vi "Igor_multi_singleXmultiY_ITX.vi"(1 "message":string, 2 "x-column name":string="field", 3 "graph file":cluster{"all rows":dbl[], "all rows":dbl[]}[](array[cluster])=[{"all rows"=array[1831 elements], "all rows"=array[1831 elements]}, {"all rows"=array[1238 elements], "all rows"=array[1238 elements]}, {"all rows"=array[1485 elements], "all rows"=array[1485 elements]}] {"all rows" format="%.2e"; "all rows" format="%.2f"}, 4 "Y-column names":string[](array[string])=["mr"], 5 "window name":string="Data1", 6 "column extension":string[](array[string])=["003", "004", "005"], 7 "file":path) -> (0 "new file path (Not A Path if cancelled)":path=path "C:/work/data/Magnet runs/Cell 9 2017 Summer School/test_window2.itx")   [LabVIEW 2020]
uses:
  <vilib>/Utility/file.llb/Write To Spreadsheet File (DBL).vi
panel:
  out "Y-column names 2":string[](array[string])
  out "String":string="\rX ModifyGraph rgb(mr_003)=(0,0,0),rgb(mr_004)=(65280,0,0),rgb(mr_005)=(0,65280,0);DelayUpdate\r"
  in  "starting commands":string="X preferences 0"
  in  "concluding commnads":string="X preferences 1\nX KillStrings S_waveNames"
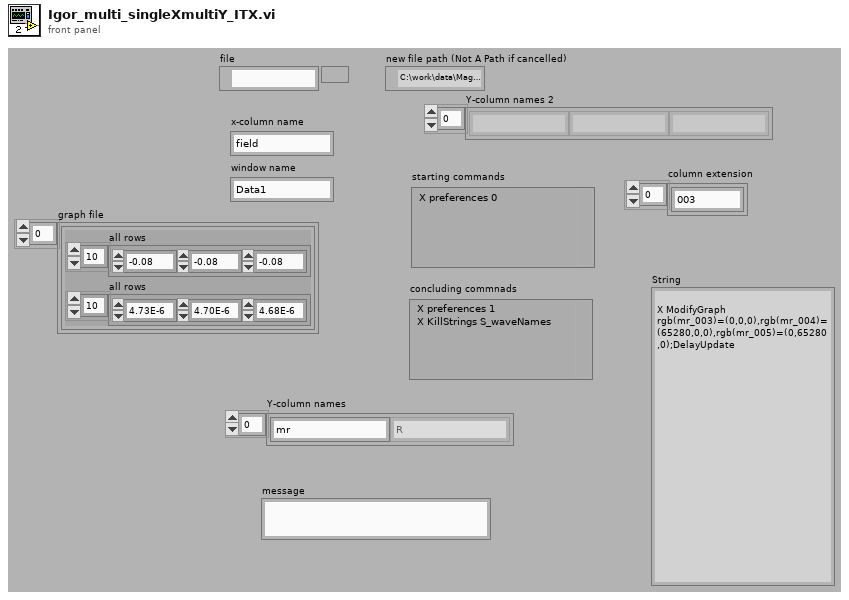
[diagram p1: front panel]
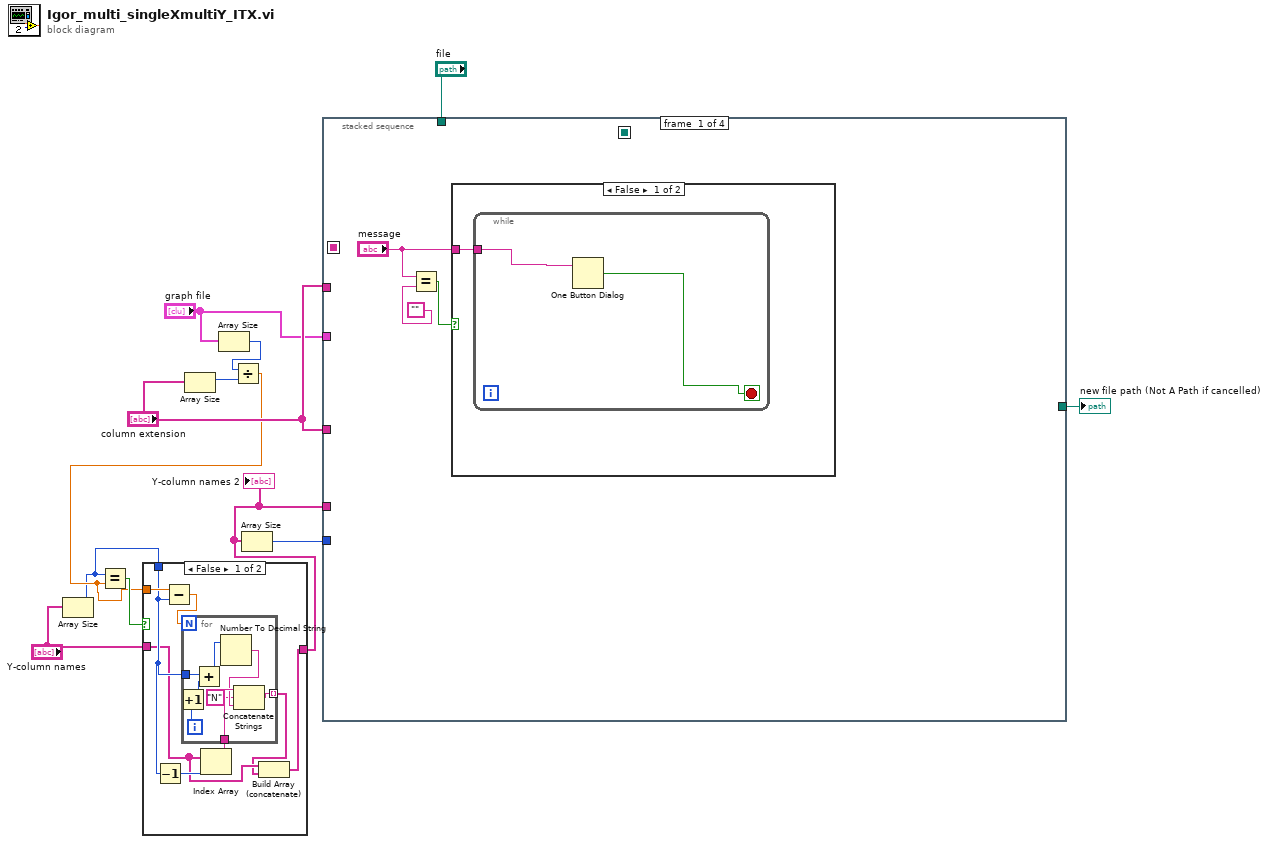
[diagram p0: block diagram]
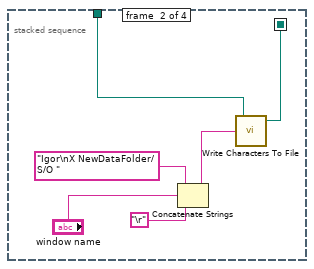
[diagram p4: hidden frame]
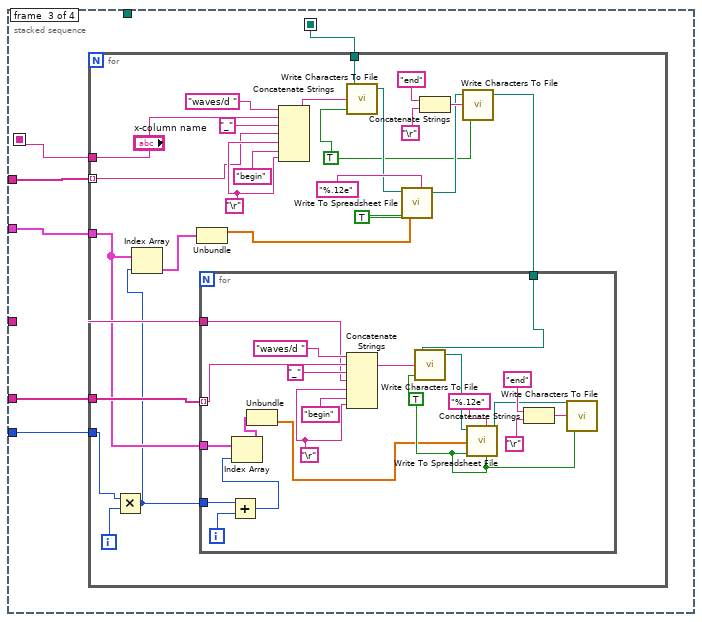
[diagram p5: hidden frame]
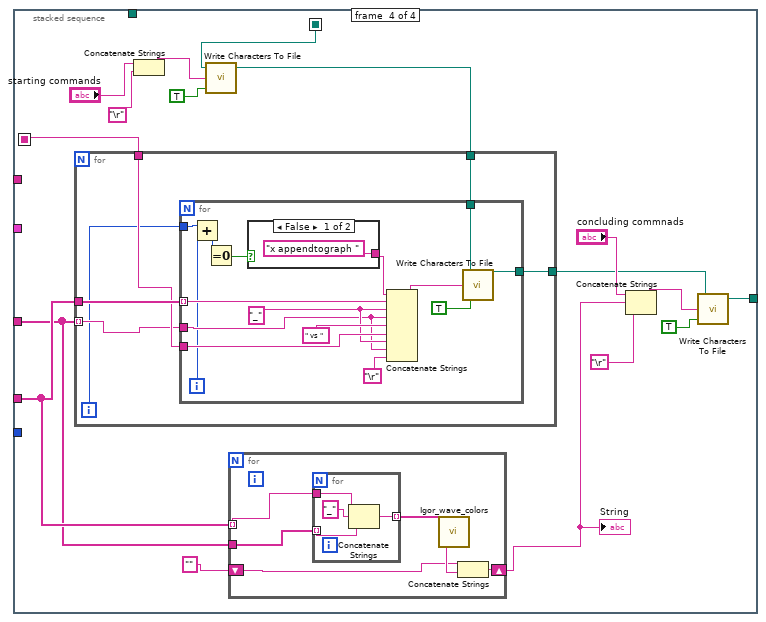
[diagram p6: hidden frame]
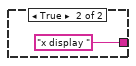
[diagram p7: hidden frame]
diagram:
  n1 = Array Size(array="Y-column names") -> (size(s)=w1:i32)
  n2 = Array Size(array="column extension") -> (size(s)=w8:i32)
  n3 = Array Size(array="graph file") -> (size(s)=w6:i32)
  n4 = Divide(x=w6, y=w8) -> (x/y=w2:dbl)
  n5 = Equal?(x=w1, y=w2) -> (x = y?=w5:bool)
  n6 = case shown="False" w5 {
    tunnel: [w15 w29] -> w3
    tunnel: "Y-column names" -> [w16 w29]
    tunnel: w2 -> [w19 _]
    tunnel: w1 -> [w18 _]
    frame False {
      n7 = Decrement(x=w18) -> (x-1=w17:i32)
      n8 = Subtract(x=w19, y=w18) -> (x-y=w20:dbl)
      n9 = Index Array(array=w16, index=w17) -> (element=w14:string)
      n10 = for {
        N: w20 -> [_]
        tunnel: w18 -> [w26]
        tunnel: w14 -> [w24]
        tunnel: [w23] -> w13 mode=indexing
        i -> [w28]
        n11 = Increment(x=w28) -> (x+1=w25:i32)
        n12 = Add(x=w26, y=w25) -> (x+y=w27:i32)
        n13 = Number To Decimal String(number=w27) -> (decimal integer string=w22:string)  [unwired: 1 in]
        n14 = Concatenate Strings(w24, "N" ("string"), w22) -> (w23:string)
      }
      n15 = Build Array (concatenate)(w16, w13) -> (w15:string[])
    }
    frame True {
    }
  }
  "Y-column names 2" <- w3
  n16 = Array Size(array=w3) -> (size(s)=w7:i32)
  n17 = stacked-sequence {
    seq-local: [_ _ w46 _] -> [_ _ _ w100]
    seq-local: [_ w36 _ _] -> [_ _ w45 w99]
    tunnel: "file" -> [_ w37 _ _]
    tunnel: "column extension" -> [_ _ w47 _]
    tunnel: "graph file" -> [_ _ w43 _]
    tunnel: "column extension" -> [_ _ _ w96]
    tunnel: [_ _ _ w98] -> w11
    tunnel: w3 -> [_ _ w44 w97]
    tunnel: w7 -> [_ _ w42 _]
    frame #0 {
      n18 = Equal?(x="message", y="") -> (x = y?=w30:bool)
      n19 = case shown="False" w30 {
        tunnel: "message" -> [w33 _]
        frame False {
          n20 = while {
            tunnel: w33 -> [w34]
            stop <- w35 stop-if-true
            n21 = One Button Dialog(message=w34) -> (true=w35:bool)  [unwired: 1 out]
          }
        }
        frame True {
        }
      }
    }
    frame #1 {
      n22 = Concatenate Strings("Igor\nX NewDataFolder/S/O " ("character string"), "window name", "\r") -> (w39:string)
      n23 = call <vilib>:"Write Characters To File.vi"("character string"=w39, "file path (dialog if empty)"=w37) -> ("new file path (Not A Path if cancelled)"=w36:path)  [unwired: 1 in, 2 out]
    }
    frame #2 {
      n24 = for {
        tunnel: w45 -> [w65]
        tunnel: w47 -> [w56] mode=indexing
        tunnel: ["x-column name"] -> w46
        tunnel: w44 -> [w53]
        tunnel: w43 -> [w49]
        tunnel: w42 -> [w52]
        i -> [w50]
        w62 = TRUE
        w66 = "\r"
        w54 = TRUE ("append to file? (new file:F)")
        n25 = Multiply(x=w52, y=w50) -> (x*y=w48:i32)
        n26 = Index Array(array=w49, index=w48) -> (element=w51:cluster{"all rows":dbl[], "all rows":dbl[]})
        n27 = Unbundle(w51) -> ("all rows"=w63:dbl[])  [unwired: 1 out]
        n28 = Concatenate Strings("waves/d ", "x-column name", "_", w56, w66, "begin", w66) -> (w68:string)
        n29 = call <vilib>:"Write Characters To File.vi"("append to file? (new file:F)"=w54, "character string"=w68, "file path (dialog if empty)"=w65) -> ("new file path (Not A Path if cancelled)"=w61:path)  [unwired: 2 out]
        n30 = call-poly <vilib>:"Write To Spreadsheet File.vi"("transpose? (no:F)"=w62, "format (%.3f)"="%.12e", "append to file? (new file:F)"=w62, "1D data"=w63, "file path (dialog if empty)"=w61) -> ("new file path (Not A Path if cancelled)"=w57:path)  [unwired: 1 in, 2 out]
        n31 = Concatenate Strings("end", "\r") -> (w58:string)
        n32 = call <vilib>:"Write Characters To File.vi"("append to file? (new file:F)"=w54, "character string"=w58, "file path (dialog if empty)"=w57) -> ("new file path (Not A Path if cancelled)"=w55:path)  [unwired: 2 out]
        n33 = for {
          tunnel: w53 -> [w87] mode=indexing
          tunnel: w56 -> [w86]
          tunnel: w55 -> [w84]
          tunnel: w48 -> [w77]
          tunnel: w49 -> [w74]
          i -> [w76]
          w88 = "\r"
          w78 = TRUE ("append to file? (new file:F)")
          n34 = Add(x=w77, y=w76) -> (x+y=w75:i32)
          n35 = Index Array(array=w74, index=w75) -> (element=w73:cluster{"all rows":dbl[], "all rows":dbl[]})
          n36 = Unbundle(w73) -> ("all rows"=w72:dbl[])  [unwired: 1 out]
          n37 = Concatenate Strings("waves/d ", w87, "_", w86, w88, "begin", w88) -> (w90:string)
          n38 = call <vilib>:"Write Characters To File.vi"("append to file? (new file:F)"=w78, "character string"=w90, "file path (dialog if empty)"=w84) -> ("new file path (Not A Path if cancelled)"=w83:path)  [unwired: 2 out]
          n39 = call-poly <vilib>:"Write To Spreadsheet File.vi"("transpose? (no:F)"=w78, "format (%.3f)"="%.12e", "append to file? (new file:F)"=w78, "1D data"=w72, "file path (dialog if empty)"=w83) -> ("new file path (Not A Path if cancelled)"=w79:path)  [unwired: 1 in, 2 out]
          n40 = Concatenate Strings("end", "\r") -> (w80:string)
          n41 = call <vilib>:"Write Characters To File.vi"("append to file? (new file:F)"=w78, "character string"=w80, "file path (dialog if empty)"=w79) -> ()  [unwired: 3 out]
        }
      }
    }
    frame #3 {
      n42 = Concatenate Strings("starting commands", "\r") -> (w107:string)
      n43 = call <vilib>:"Write Characters To File.vi"("append to file? (new file:F)"=TRUE, "character string"=w107, "file path (dialog if empty)"=w99) -> ("new file path (Not A Path if cancelled)"=w106:path)  [unwired: 2 out]
      n44 = for {
        tunnel: w106 -> [w125]
        tunnel: [w124] -> w102
        tunnel: w100 -> [w122]
        tunnel: w96 -> [w121] mode=indexing
        tunnel: w97 -> [w123]
        i -> [w120]
        n45 = for {
          tunnel: w125 -> [w140]
          tunnel: [w139] -> w124
          tunnel: w123 -> [w138] mode=indexing
          tunnel: w122 -> [w137]
          tunnel: w121 -> [w129]
          tunnel: w120 -> [w127]
          i -> [w128]
          w132 = "_"
          n46 = Add(x=w127, y=w128) -> (x+y=w126:i32)
          n47 = Equal To 0?(x=w126) -> (x = 0?=w130:bool)
          n48 = case shown="False" w130 {
            tunnel: ["x appendtograph " "x display "] -> w134
            frame False {
            }
            frame True {
            }
          }
          n49 = Concatenate Strings(w134, w138, w132, w129, " vs ", w137, w132, w129, "\r") -> (w136:string)
          n50 = call <vilib>:"Write Characters To File.vi"("append to file? (new file:F)"=TRUE, "character string"=w136, "file path (dialog if empty)"=w140) -> ("new file path (Not A Path if cancelled)"=w139:path)  [unwired: 2 out]
        }
      }
      n51 = for {
        tunnel: w96 -> [w114]
        tunnel: w97 -> [w115] mode=indexing
        shift-right: [w112] -> w93
        shift-left: "" -> [w110]
        n52 = for {
          tunnel: w115 -> [w118]
          tunnel: [w117] -> w113 mode=indexing
          tunnel: w114 -> [w116] mode=indexing
          n53 = Concatenate Strings(w118, "_", w116) -> (w117:string)
        }
        n54 = call "Igor_wave_colors.vi"("Array"=w113) -> ("concatenated string"=w111:string)
        n55 = Concatenate Strings(w110, w111) -> (w112:string)
      }
      "String" <- w93
      n56 = Concatenate Strings("concluding commnads", w93, "\r") -> (w103:string)
      n57 = call <vilib>:"Write Characters To File.vi"("append to file? (new file:F)"=TRUE, "character string"=w103, "file path (dialog if empty)"=w102) -> ("new file path (Not A Path if cancelled)"=w98:path)  [unwired: 2 out]
    }
  }
  "new file path (Not A Path if cancelled)" <- w11
